vi "To String.vi"(8 "error in (no error)":errorcluster, 11 "Types in":refnum<class "Abs_Boolean_1D.lvclass">) -> (0 "error out":errorcluster, 2 "String":string, 3 "Types out":refnum<class "Abs_Boolean_1D.lvclass">)   [LabVIEW 2021, in "Abs_Boolean_1D.lvclass"]
uses:
  Abs_Boolean_1D.lvclass
  Abs_Boolean_1D.lvclass/Abs_Boolean_1D.ctl
  Properties/Read To String_True.vi
  Properties/Read To String_False.vi
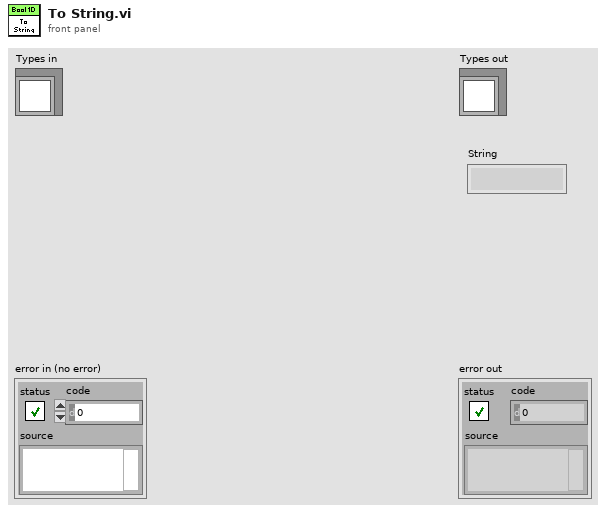
[diagram p1: front panel]
types:
  T1 = typedef "Abs_Boolean_1D.lvclass/Element Type.ctl" = bool
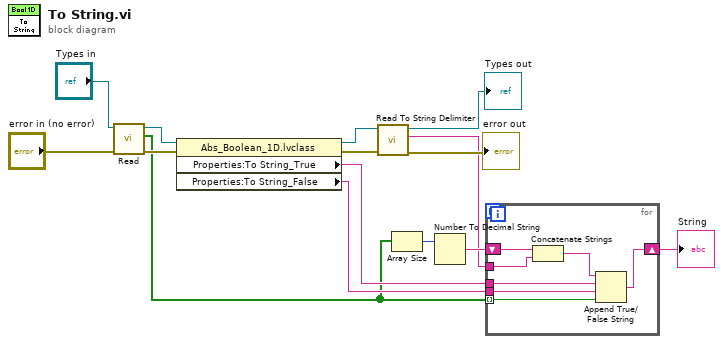
[diagram p0: block diagram]
diagram:
  n1 = call-dynamic "Read.vi"("error in (no error)"="error in (no error)", "Boolean in"="Types in") -> ("error out"=w13:errorcluster, "Boolean 1D"=w6:T1[], "Boolean out"=w12:refnum<class "Abs_Boolean_1D.lvclass">)  [unwired: 7 in]
  n2 = property class="Abs_Boolean_1D.lvclass"(reference=w12, error in=w13) -> (reference out=w4:refnum<class "Abs_Boolean_1D.lvclass">, error out=w5:errorcluster, "Properties:To String_True"=w11:string, "Properties:To String_False"=w10:string)
  n3 = call-dynamic "Read To String Delimiter.vi"("error in (no error)"=w5, "Abs_Array in"=w4) -> ("error out"=→"error out":errorcluster, "To String Delimiter"=w1:string, "Abs_Array out"=→"Types out":refnum<class "Abs_Boolean_1D.lvclass">)  [unwired: 7 in]
  n4 = Array Size(array=w6) -> (size(s)=w7:i32)
  n5 = Number To Decimal String(number=w7) -> (decimal integer string=w8:string)  [unwired: 1 in]
  n6 = for {
    tunnel: w11 -> [w22]
    tunnel: w10 -> [w21]
    shift-right: [w20] -> w9
    shift-left: w8 -> [w18]
    tunnel: w6 -> [w19] mode=indexing
    tunnel: w1 -> [w16]
    n7 = Concatenate Strings(w18, w16) -> (w17:string)
    n8 = Append True/False String(1:w19, 2:w21, 3:w22, 4:w17) -> (0:w20:string)
  }
  "String" <- w9
